vi "FatorDePasseStriker.vi"(6 "atacando ao contrário?":bool=TRUE, 8 "Função":T1, 9 "id":u32, 10 "IA State Input":T3={"our_robots"=[], "enemy_robots"=[], "balls"=[], "geometry"={"line_width"=0, "field_length"=0, "field_width"=0, "boundary_width"=0, "referee_width"=0, "goal_width"=0, "goal_depth"=0, "goal_wall_width"=0, "center_circle_radius"=0, "defense_radius"=0, "defense_stretch"=0, "free_kick_from_defense_dist"=0, "penalty_spot_from_field_line_dist"=0, "penalty_line_from_spot_dist"=0}, "IA Judge"={"stage"="", "command"="", "our_goalie_id"=0.0, "enemy_goalie_id"=0.0, "command enum"=enum."Halt", "Time"=enum."Azul"}, "Received Timestamp"=timestamp(0 s since 1904-01-01), "Events"={"Touch"=FALSE, "Ball out"=FALSE, "id touch"=0.0, "Ball out of \nVision"=FALSE, "Ball inside \nGoalie area"=FALSE, "Robot not responding"=FALSE, "Robots responding status"=[1.0, 1.0, 1.0, 1.0, 1.0, 1.0], "Enemy Ball \nPossession"=FALSE, "Pass State"=FALSE, "id end of pass"=0.0, "Kick"=FALSE, "Id ini Possession"=0.0, "Ball Possesion"=FALSE, "Id Possesion"=0.0, "Direct Kick"=FALSE, "2nd Strk Ativo"=FALSE}}, 11 "AI Parameters":T2={"GotoKick"={"Dist do cone a frente"=150.0, "attacker farback"=1500.0, "Perto"=300.0, "min dist to kick"=150.0, "kick eps"=0.0, "Time to transition"=0.05}, "Attacker"={"CC chute"=0.09, "CC passe"=0.045, "Kick Force"=100.0, "ball-robot Kick"=200.0, "ball-robot Pass"=0.3, "drible\nAttk"=FALSE}, "Defender"={"D max"=1700.0, "Vel p/ robô av"=1000.0, "Kick Force"=100.0, "D atk-def"=0.0, "D farback"=0.0, "drible\ndef"=FALSE, "drible\ngoalie"=FALSE}, "Timeout"={"Field/v in x"=6.0, "Dist Robots"=300, "Dist up in y"=300}, "Pose Striker"={"dist"=200.0, "Numeric"=-4.0, "dist 2"=200.0, "drible\nstriker"=FALSE}, "Dist Stop"=300.0, "D ball out"=200, "D central gap "=150.0, "T pass"=0.0, "Force ++"=0.0, "range kick"=0.0, "Chute alto"=TRUE, "Marcador novo"=TRUE, "drible"=FALSE, "D drible"=300.0, "Versão Striker"=enum."3", "Defesa"=enum."ManMark", "Marcador"=enum."Marcar Segundo mais perigoso", "Receptor passe"=enum."2nd Striker", "Área"=enum."Quadrada", "Decisão\nsimples?"=FALSE} {"D drible" format="%#_13g"; "D central gap" format="%#_13g"; "Dist Stop" format="%#_13g"; "Pose Striker"."Numeric" format="%#_13g"; "Defender"."Kick Force" format="%#_13g"; "Defender"."Vel p/ robô av" format="%#_13g"; "Attacker"."ball-robot Kick" format="%#_13g"; "Attacker"."Kick Force" format="%#_13g"; "Attacker"."CC passe" format="%#_13g"; "Attacker"."CC chute" format="%#_13g"; "GotoKick"."kick eps" format="%#_13g"; "GotoKick"."min dist to kick" format="%#_13g"; "GotoKick"."Perto" format="%#_13g"; "GotoKick"."attacker farback" format="%#_13g"; "GotoKick"."Dist do cone a frente" format="%#_13g"}) -> (1 "Fator de passe":dbl, 2 "Dif. tempo\ninimigo bola":dbl, 3 "Robô marcado?":bool=TRUE, 7 "menor dist":dbl)   [LabVIEW 2018]
uses:
  Core/AI Input.ctl
  Core/AI Robot.ctl
  Functions Enum.ctl
  AttackerStates.ctl
  Path Planning/RRT/PathDests.ctl
  Path Planning/RRT/PathDest.ctl
  Core/AI Ball.ctl
  Core/Field Size.ctl
  Core/AI Judge.ctl
  Command Enum.ctl
  Util/Events/Events.ctl
  AI Parameters.ctl
  d3ae8bea-2540-4cab-b848-3da8b8f91e54.vi
  <vilib>/Array/Sort 2D Array - Pop Stack.vi
  <vilib>/Array/Sort 2D Array - Push Stack.vi
panel:
  out "Critério de marcação Normalizado":dbl
  out "Goal Gap Normalizado(%do gol aberta)":dbl
  out "id inimigo \nmaior diferença \nde tempo":dbl
  out "Array":dbl[][](array[numeric])
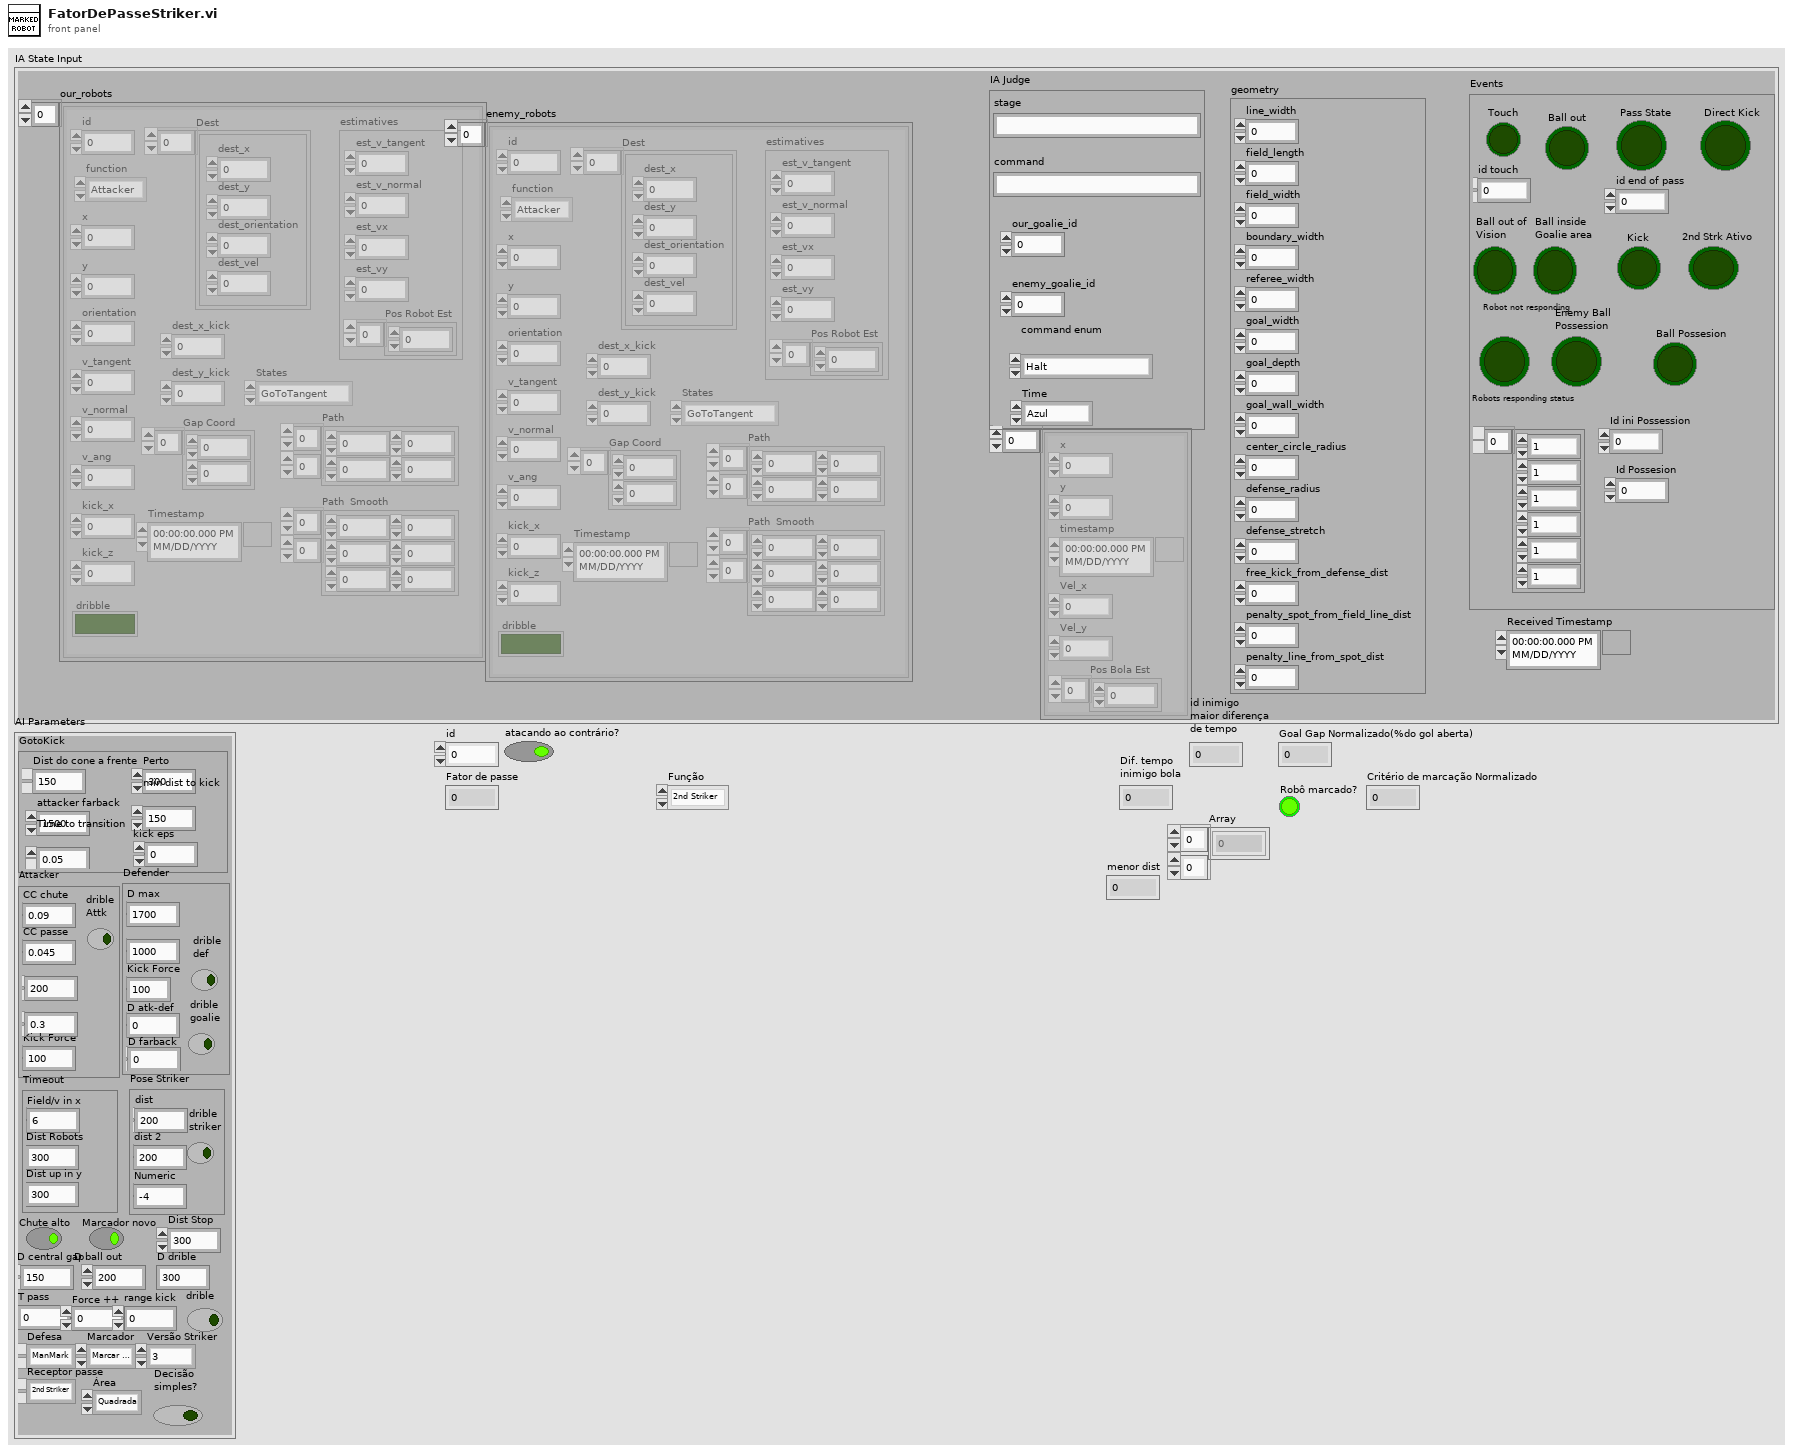
[diagram p1: front panel]
types:
  T1 = typedef "Functions Enum.ctl" = enum16{"2nd Striker", "Attacker", "Goalie", "Defender", "Striker", "Goto 0", "Dummy", "Kicker", "ZigZag 0", "ZigZag 1", "ZigZag 2", "ZigZag 3", "ZigZag 4", "ZigZag 5", "ZigZag 6", "ZigZag 7", "ZigZag 8", ""}
  T2 = typedef "AI Parameters.ctl" = cluster{"GotoKick":cluster{"Dist do cone a frente":dbl, "attacker farback":dbl, "Perto":dbl, "min dist to kick":dbl, "kick eps":dbl, "Time to transition":dbl}, "Attacker":cluster{"CC chute":dbl, "CC passe":dbl, "Kick Force":dbl, "ball-robot Kick":dbl, "ball-robot Pass":dbl, "drible\nAttk":bool}, "Defender":cluster{"D max":dbl, "Vel p/ robô av":dbl, "Kick Force":dbl, "D atk-def":dbl, "D farback":dbl, "drible\ndef":bool, "drible\ngoalie":bool}, "Timeout":cluster{"Field/v in x":dbl, "Dist Robots":u32, "Dist up in y":u32}, "Pose Striker":cluster{"dist":dbl, "Numeric":dbl, "dist 2":dbl, "drible\nstriker":bool}, "Dist Stop":dbl, "D ball out":i32, "D central gap ":dbl, "T pass":dbl, "Force ++":dbl, "range kick":dbl, "Chute alto":bool, "Marcador novo":bool, "drible":bool, "D drible":dbl, "Versão Striker":enum16{"Auto", "3", "2", "1"}, "Defesa":enum16{"ManMark", "Barreira"}, "Marcador":enum16{"Marcar Segundo mais perigoso", "Marcar o mais perigoso"}, "Receptor passe":enum16{"Auto", "2nd Striker", "Striker"}, "Área":enum16{"Quadrada", "Circular"}, "Decisão\nsimples?":bool}
  T3 = typedef "AI Input.ctl" = cluster{"our_robots":T4[], "enemy_robots":T4[], "balls":T8[], "geometry":T9, "IA Judge":T10, "Received Timestamp":timestamp, "Events":T12}
  T4 = typedef "AI Robot.ctl" = cluster{"id":u32, "function":T1, "x":dbl, "y":dbl, "orientation":dbl, "v_tangent":dbl, "v_normal":dbl, "v_ang":dbl, "kick_x":dbl, "kick_z":dbl, "dribble":bool, "Timestamp":timestamp, "estimatives":cluster{"est_v_tangent":dbl, "est_v_normal":dbl, "est_vx":dbl, "est_vy":dbl, "Pos Robot Est":dbl[]}, "dest_x_kick":dbl, "dest_y_kick":dbl, "Gap Coord":dbl[], "States":T5, "Path ":dbl[][], "Path  Smooth":dbl[][], "Dest":T6}
  T5 = typedef "AttackerStates.ctl" = enum16{"Pass", "GoToTangent", "BallGetting", "GoToKick", ""}
  T6 = typedef "PathDests.ctl" = T7[]
  T7 = typedef "PathDest.ctl" = cluster{"dest_x":dbl, "dest_y":dbl, "dest_orientation":dbl, "dest_vel":dbl}
  T8 = typedef "AI Ball.ctl" = cluster{"x":dbl, "y":dbl, "timestamp":timestamp, "Vel_x":dbl, "Vel_y":dbl, "Pos Bola Est":dbl[]}
  T9 = typedef "Field Size.ctl" = cluster{"line_width":u32, "field_length":u32, "field_width":u32, "boundary_width":u32, "referee_width":u32, "goal_width":u32, "goal_depth":u32, "goal_wall_width":u32, "center_circle_radius":u32, "defense_radius":u32, "defense_stretch":u32, "free_kick_from_defense_dist":u32, "penalty_spot_from_field_line_dist":u32, "penalty_line_from_spot_dist":u32}
  T10 = typedef "AI Judge.ctl" = cluster{"stage":string, "command":string, "our_goalie_id":dbl, "enemy_goalie_id":dbl, "command enum":T11, "Time":enum16{"Azul", "Amarelo"}}
  T11 = typedef "Command Enum.ctl" = enum16{"Halt", "Stop", "Force Start", "PKA Normal Start", "Prepare Kickoff Ally", "PKE Normal Start", "Prepare Kickoff Enemy", "Prepare Penalty Ally", "PPA Normal Start", "Prepare Penalty Enemy", "PPE Normal Start", "Direct Free Enemy", "Direct Free Ally", "Indirect Free Enemy", "Indirect Free Ally", "Timeout Enemy", "Timeout Ally", "Goal Enemy", "Goal Ally", "Ball Placement Enemy", "Ball Placement Ally", "Normal Half Time", "Extra Time Break", "Extra Half Time", "None", "Post Game"}
  T12 = typedef "Events.ctl" = cluster{"Touch":bool, "Ball out":bool, "id touch":dbl, "Ball out of \nVision":bool, "Ball inside \nGoalie area":bool, "Robot not responding":bool, "Robots responding status":dbl[], "Enemy Ball \nPossession":bool, "Pass State":bool, "id end of pass":dbl, "Kick":bool, "Id ini Possession":dbl, "Ball Possesion":bool, "Id Possesion":dbl, "Direct Kick":bool, "2nd Strk Ativo":bool}
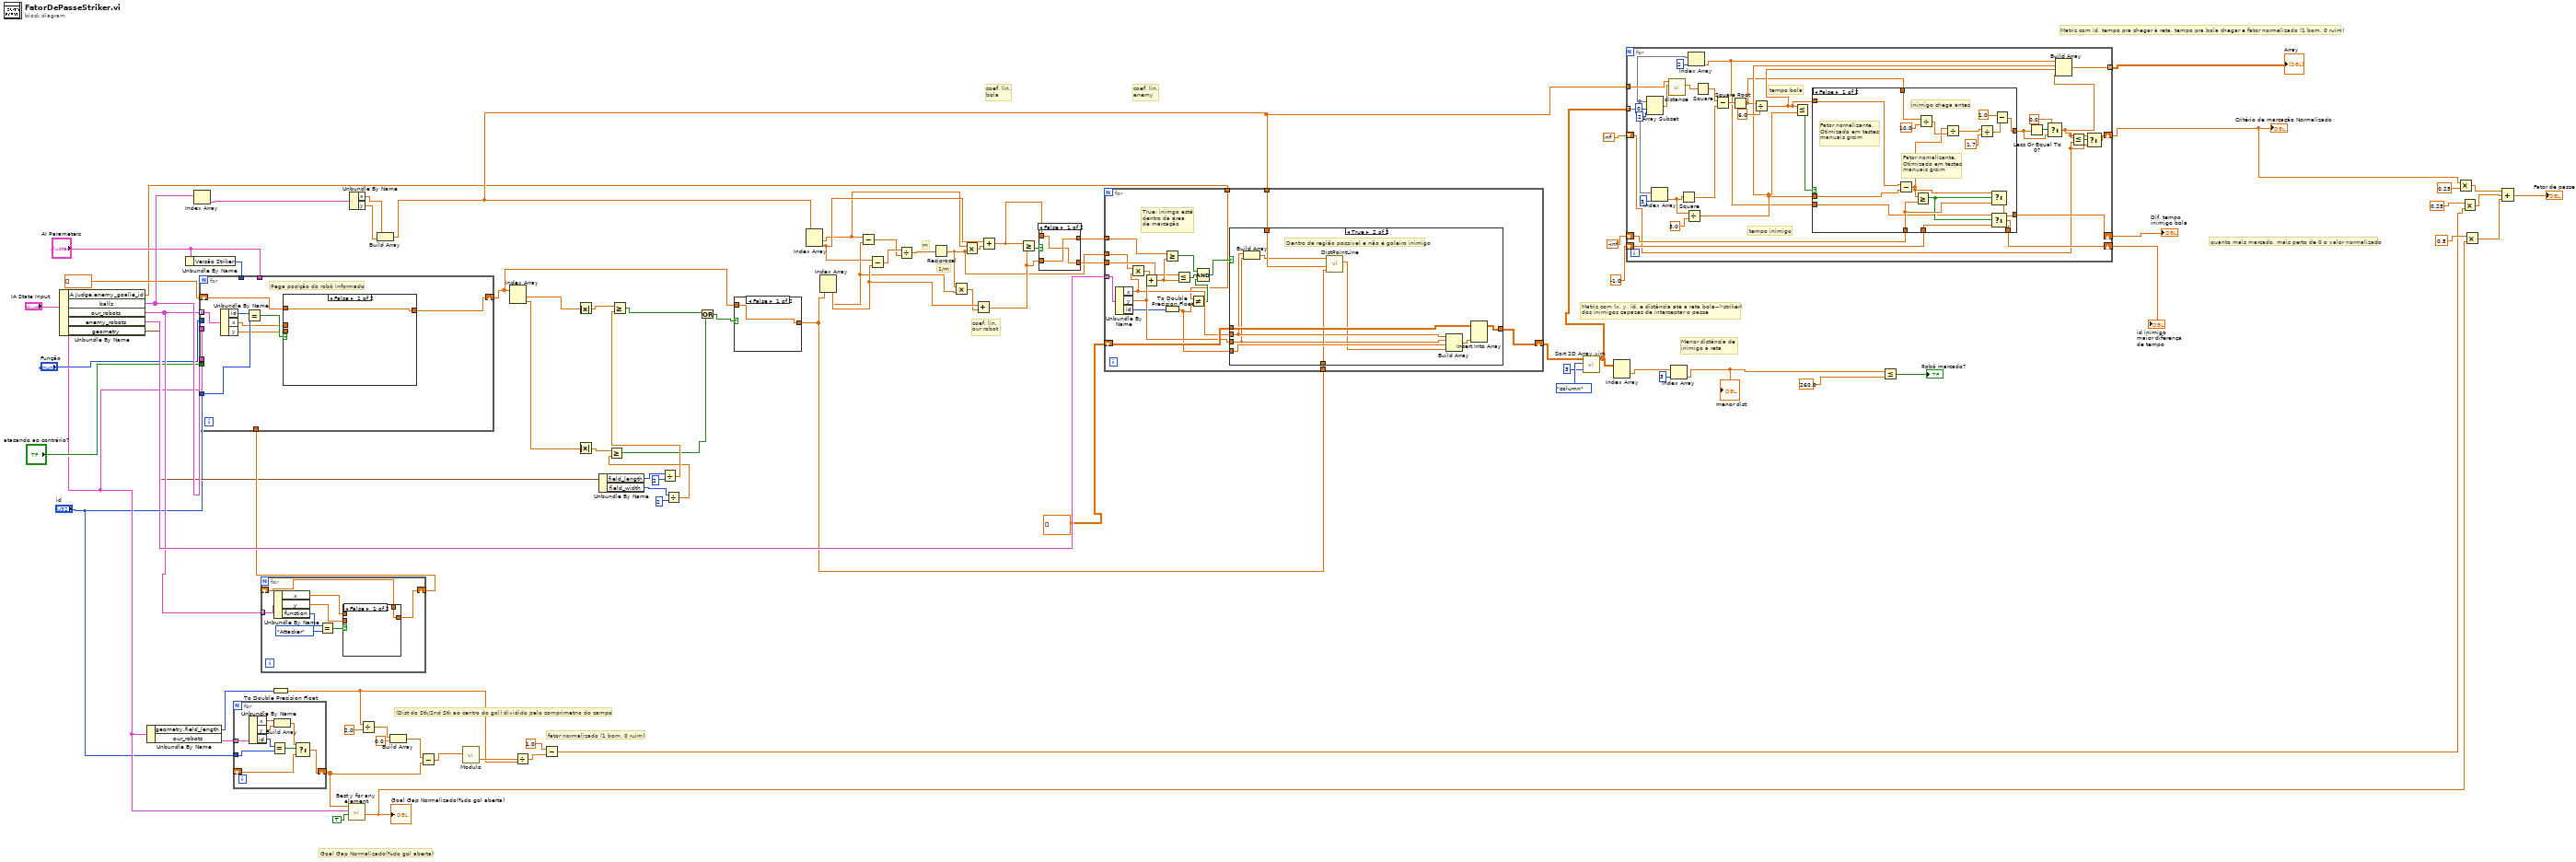
[diagram p0: block diagram]
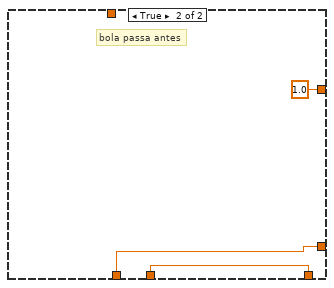
[diagram p2: hidden frame]
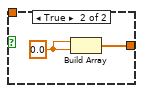
[diagram p3: hidden frame]
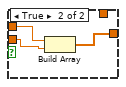
[diagram p4: hidden frame]
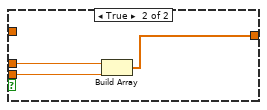
[diagram p7: hidden frame]
diagram:
  # "Goal Gap Normalizado(%do gol aberta)"
  # "fator normalizado (1 bom, 0 ruim)"
  # "(Dist do Stk/2nd Stk ao centro do gol) dividido pelo comprimetno do campo"
  # "Matriz com id, tempo pra chegar à reta, tempo pra bola chegar e fator normalizado (1 bom, 0 ruim)"
  # "quanto mais marcado, mais perto de 0 o valor normalizado"
  # "Menor distância de \ninimigo à reta"
  # "Matriz com (x, y, id, e distância até a reta bola-->striker) \ndos inimigos capazes de interceptar o passe"
  # "coef. lin.\nbola"
  # "coef. lin.\nenemy"
  # "coef. lin.\nour robot"
  # "1/m"
  # "m"
  n1 = Unbundle By Name("IA State Input") -> ("IA Judge.enemy_goalie_id"=w23:dbl, "balls"=w65:T8[], "our_robots"=w64:T4[], "enemy_robots"=w78:T4[], "geometry"=w52:T9)
  n2 = Unbundle By Name("IA State Input") -> ("geometry.field_length"=w18:u32, "our_robots"=w27:T4[])
  n3 = Unbundle By Name("AI Parameters") -> ("Versão Striker"=w47:enum16{"Auto", "3", "2", "1"})
  n4 = Index Array(array=w65) -> (element=w86:T8)  [unwired: 1 in]
  n5 = for {
    tunnel: w27 -> [w95] mode=indexing
    tunnel: "id" -> [w93]
    shift-right: [w89] -> w16
    shift-left: _ -> [w87]
    n6 = Unbundle By Name(w95) -> ("x"=w92:dbl, "y"=w91:dbl, "id"=w94:u32)
    n7 = Equal?(x=w94, y=w93) -> (x = y?=w88:bool)
    n8 = Build Array(w92, w91) -> (w90:dbl[])
    n9 = Select(t=w90, s=w88, f=w87) -> (s? t:f=w89:dbl[])
  }
  n10 = for {
    tunnel: w64 -> [w103] mode=indexing
    shift-right: [w97] -> w63
    shift-left: _ -> [w96]
    n11 = Unbundle By Name(w103) -> ("x"=w99:dbl, "y"=w98:dbl, "function"=w102:T1)
    n12 = Equal?(x=w102, y=Functions_Enum."Attacker") -> (x = y?=w100:bool)
    n13 = case shown="False" w100 {
      tunnel: w99 -> [_ w107]
      tunnel: w98 -> [_ w106]
      tunnel: [w104 w105] -> w97
      tunnel: w96 -> [w104 _]
      frame False {
      }
      frame True {
        n14 = Build Array(w107, w106) -> (w105:dbl[])
      }
    }
  }
  n15 = for {
    tunnel: w64 -> [w115] mode=indexing
    tunnel: "id" -> [w113]
    shift-right: [w109] -> w29
    shift-left: dbl[] [] -> [w108]
    tunnel: "IA State Input" -> [_]
    tunnel: w65 -> [_]
    tunnel: "AI Parameters" -> [_]
    tunnel: w63 -> [_]
    tunnel: "Função" -> [_]
    tunnel: w47 -> [_]
    tunnel: "atacando ao contrário?" -> [_]
    # "Pega posição do robô informado"
    n16 = Unbundle By Name(w115) -> ("id"=w114:u32, "x"=w111:dbl, "y"=w110:dbl)
    n17 = Equal?(x=w114, y=w113) -> (x = y?=w112:bool)
    n18 = case shown="False" w112 {
      tunnel: w111 -> [_ w119]
      tunnel: w110 -> [_ w118]
      tunnel: [w116 w117] -> w109
      tunnel: w108 -> [w116 _]
      frame False {
      }
      frame True {
        n19 = Build Array(w119, w118) -> (w117:dbl[])
      }
    }
  }
  n20 = To Double Precision Float(number=w18) -> (double precision float=w2:dbl)
  n21 = call "Best y for any element.vi"("Maior intervalo(T)\nMaior angulo(F)"=TRUE ("Maior intervalo(T)\nMaior angulo(F)"), "IA State"="IA State Input", "Element Position"=w16) -> ("Goal Gap Normalizado(%do gol aberta)"=w11:dbl)  [unwired: 4 in, 4 out]
  "Goal Gap Normalizado(%do gol aberta)" <- w11
  n22 = Unbundle By Name(w86) -> ("x"=w85:dbl, "y"=w84:dbl)
  n23 = Divide(x=w2, y=2.0) -> (x/y=w20:dbl)
  n24 = Build Array(w85, w84) -> (w43:dbl[])
  n25 = Build Array(w20, 0.0 ("element")) -> (w17:dbl[])
  n26 = Subtract(x=w17, y=w16) -> (x-y=w15:dbl[])
  n27 = call "Modulo.vi"("2D vector"=w15) -> ("Modulo"=w4:dbl)  [unwired: 10 in]
  n28 = Index Array(array=w29) -> (element #1=w31:dbl, element #2=w30:dbl)  [unwired: 2 in]
  n29 = Divide(x=w4, y=w2) -> (x/y=w3:dbl)
  n30 = Subtract(x=1.0, y=w3) -> (x-y=w1:dbl)
  n31 = Absolute Value(x=w31) -> (abs(x)=w58:dbl)
  n32 = Absolute Value(x=w30) -> (abs(x)=w56:dbl)
  n33 = Unbundle By Name(w52) -> ("field_length"=w62:u32, "field_width"=w59:u32)
  n34 = Divide(x=w62, y=2) -> (x/y=w57:dbl)
  n35 = Greater Or Equal?(x=w58, y=w57) -> (x >= y?=w54:bool)
  n36 = Divide(x=w59, y=u32 2) -> (x/y=w55:dbl)
  n37 = Greater Or Equal?(x=w56, y=w55) -> (x >= y?=w53:bool)
  n38 = Or(x=w54, y=w53) -> (x .or. y?=w51:bool)
  n39 = case shown="False" w51 {
    tunnel: [w120 w121] -> w50
    tunnel: w29 -> [w120 _]
    frame False {
    }
    frame True {
      w122 = 0.0
      n40 = Build Array(w122, w122) -> (w121:dbl[])
    }
  }
  n41 = Index Array(array=w43) -> (element #1=w35:dbl, element #2=w82:dbl)  [unwired: 2 in]
  n42 = Index Array(array=w50) -> (element #1=w36:dbl, element #2=w81:dbl)  [unwired: 2 in]
  n43 = Subtract(x=w35, y=w36) -> (x-y=w79:dbl)
  n44 = Subtract(x=w82, y=w81) -> (x-y=w80:dbl)
  n45 = Divide(x=w80, y=w79) -> (x/y=w83:dbl)
  n46 = Reciprocal(x=w83) -> (1/x=w33:dbl)
  n47 = Multiply(x=w33, y=w36) -> (x*y=w37:dbl)
  n48 = Multiply(x=w35, y=w33) -> (x*y=w34:dbl)
  n49 = Add(x=w81, y=w37) -> (x+y=w75:dbl)
  n50 = Add(x=w82, y=w34) -> (x+y=w76:dbl)
  n51 = Greater Or Equal?(x=w76, y=w75) -> (x >= y?=w77:bool)
  n52 = case shown="False" w77 {
    tunnel: [w124 w126] -> w74
    tunnel: w76 -> [w123 w126]
    tunnel: [w123 w125] -> w73
    tunnel: w75 -> [w124 w125]
    frame False {
    }
    frame True {
    }
  }
  n53 = for {
    tunnel: w78 -> [w145] mode=indexing
    tunnel: w33 -> [w133]
    shift-right: [w143] -> w70
    shift-left: dbl[][] [] -> [w144]
    tunnel: w74 -> [w138]
    tunnel: w73 -> [w137]
    tunnel: w43 -> [w135]
    tunnel: w50 -> [w134]
    tunnel: w23 -> [w128]
    # "True: inimgo está \ndentro da área\nde marcação"
    n54 = Unbundle By Name(w145) -> ("x"=w132:dbl, "y"=w136:dbl, "id"=w130:u32)
    n55 = Multiply(x=w133, y=w132) -> (x*y=w131:dbl)
    n56 = Add(x=w131, y=w136) -> (x+y=w142:dbl)
    n57 = Greater Or Equal?(x=w138, y=w142) -> (x >= y?=w140:bool)
    n58 = To Double Precision Float(number=w130) -> (double precision float=w127:dbl)
    n59 = Less Or Equal?(x=w137, y=w142) -> (x <= y?=w141:bool)
    n60 = Not Equal?(x=w128, y=w127) -> (x != y?=w129:bool)
    n61 = Compound Arithmetic op=AND(w140, w141, w129) -> (w139:bool)
    n62 = case shown="True" w139 {
      tunnel: w144 -> [w146 w156]
      tunnel: [w146 w155] -> w143
      tunnel: w132 -> [_ w150]
      tunnel: w136 -> [_ w149]
      tunnel: w127 -> [_ w154]
      tunnel: w135 -> [_ w152]
      tunnel: w134 -> [_ w151]
      frame False {
        # "Fora da região possível ou é goleiro inimigo"
      }
      frame True {
        # "Dentro da região possível e não é goleiro inimigo"
        n63 = Build Array(w150, w149) -> (w148:dbl[])
        n64 = call "DistPointLine.vi"("P2"=w151, "P1"=w152, "Q"=w148) -> ("distance"=w147:dbl)  [unwired: 8 in]
        n65 = Build Array(w150, w149, w154, w147) -> (w153:dbl[])
        n66 = Insert Into Array(array=w156, new element=w153) -> (w155:dbl[][])  [unwired: 2 in]
      }
    }
  }
  n67 = call "Sort 2D Array.vim"("index"=3, "dimension to index (column)"=enum16{"column", "row"}."column", "2D array"=w70) -> ("sorted 2D array"=w42:dbl[][])  [unwired: 7 in, 1 out]
  n68 = Index Array(array=w42) -> (element=w44:dbl[])  [unwired: 2 in]
  n69 = for {
    tunnel: w43 -> [w170]
    tunnel: w42 -> [w169] mode=indexing
    shift-right: [w165] -> w24
    shift-left: -inf -> [w175]
    tunnel: [w174] -> w40 mode=indexing
    shift-right: [w168] -> w38
    shift-left: -1.0 ("Numeric") -> [w166]
    shift-right: [w158] -> w14
    shift-left: inf -> [w157]
    # "tempo inimigo"
    # "tempo bola"
    n70 = Array Subset(array=w169, index=0, length=2) -> (w184:dbl[])
    n71 = Index Array(array=w169, index=3) -> (element=w178:dbl)
    n72 = call "distance.vi"("P1"=w184, "P2"=w170) -> ("Dist P1P2"=w183:dbl)  [unwired: 9 in]
    n73 = Square(x=w178) -> (x^2=w181:dbl)
    n74 = Divide(x=w178, y=3.0) -> (x/y=w172:dbl)
    n75 = Index Array(array=w169, index=2) -> (element=w167:dbl)
    n76 = Square(x=w183) -> (x^2=w182:dbl)
    n77 = Subtract(x=w182, y=w181) -> (x-y=w180:dbl)
    n78 = Square Root(x=w180) -> (sqrt(x)=w164:dbl)
    n79 = Divide(x=w164, y=6.0) -> (x/y=w173:dbl)
    n80 = Less Or Equal?(x=w173, y=w172) -> (x <= y?=w176:bool)
    n81 = case shown="False" w176 {
      tunnel: w172 -> [w202 _]
      tunnel: w173 -> [w203 _]
      tunnel: [w194 w207] -> w165
      tunnel: w175 -> [w204 w207]
      tunnel: [w200 w206] -> w168
      tunnel: w167 -> [w199 _]
      tunnel: w166 -> [w198 w206]
      tunnel: w164 -> [w197 _]
      tunnel: [w189 1.0] -> w162
      frame False {
        # "Fator nomalizante.\nOtimizado em testes\nmanuais grsim"
        # "Fator nomalizante.\nOtimizado em testes\nmanuais grsim"
        # "inimigo chega antes"
        n82 = Subtract(x=w203, y=w202) -> (x-y=w188:dbl)
        n83 = Greater Or Equal?(x=w188, y=w204) -> (x >= y?=w201:bool)
        n84 = Divide(x=w197, y=10.0) -> (x/y=w195:dbl)
        n85 = Divide(x=w188, y=w195) -> (x/y=w193:dbl)
        n86 = Divide(x=w193, y=1.7) -> (x/y=w190:dbl)
        n87 = Select(t=w188, s=w201, f=w204) -> (s? t:f=w194:dbl)
        n88 = Select(t=w199, s=w201, f=w198) -> (s? t:f=w200:dbl)
        n89 = Subtract(x=1.0, y=w190) -> (x-y=w189:dbl)
      }
      frame True {
        # "bola passa antes"
      }
    }
    n90 = Less Or Equal To 0?(x=w162) -> (x <= 0?=w163:bool)
    n91 = Select(t=0.0, s=w163, f=w162) -> (s? t:f=w159:dbl)
    n92 = Build Array(w167, w172, w173, w159) -> (w174:dbl[])
    n93 = Less Or Equal?(x=w159, y=w157) -> (x <= y?=w160:bool)
    n94 = Select(t=w159, s=w160, f=w157) -> (s? t:f=w158:dbl)
  }
  "Dif. tempo\ninimigo bola" <- w24
  "Array" <- w40
  "id inimigo \nmaior diferença \nde tempo" <- w38
  "Critério de marcação Normalizado" <- w14
  n95 = Index Array(array=w44, index=3) -> (element=w45:dbl)
  "menor dist" <- w45
  n96 = Less Or Equal?(x=w45, y=260.0) -> (x <= y?=→"Robô marcado?":bool)
  n97 = Multiply(x=w14, y=0.25) -> (x*y=w13:dbl)
  n98 = Multiply(x=0.25 ("y"), y=w1) -> (x*y=w12:dbl)
  n99 = Multiply(x=0.5 ("y"), y=w11) -> (x*y=w10:dbl)
  n100 = Compound Arithmetic op=ADD(w13, w12, w10) -> (→"Fator de passe":dbl)
